vi "VL53L0X_PerformRefCalibration.vi"(11 "REV2mDistanceSensorDevRef":T1) -> (1 "PhaseCal":u8, 2 "VhvSettings":u8, 3 "REV2mDistanceSensorDevRef Out":T1)   [LabVIEW 2019, in "DistanceSensorDriver.lvlib"]
uses:
  DistanceSensorDriver.lvlib
  Typedef/REV2mDistanceSensorDevRef.ctl
  Typedef/Ports.ctl
panel:
  in  "PhaseCal":u8
  in  "VhvSettings":u8
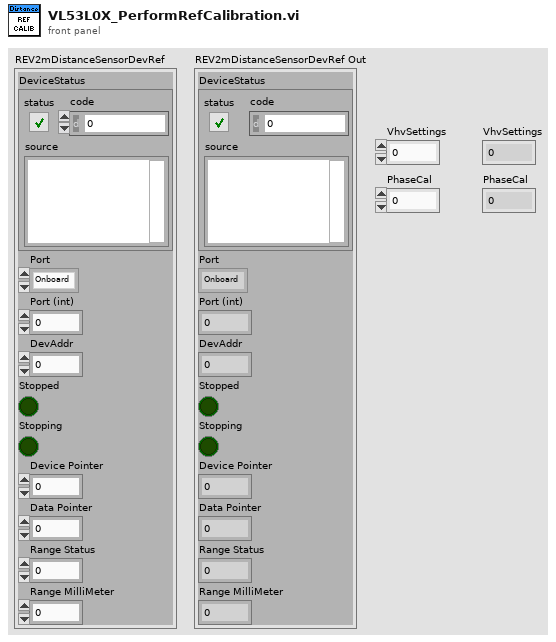
[diagram p1: front panel]
types:
  T1 = typedef "DistanceSensorDriver.lvlib/REV2mDistanceSensorDevRef.ctl" = cluster{"DeviceStatus":errorcluster, "Port":T2, "Port (int)":i32, "DevAddr":i32, "Stopped":bool, "Stopping":bool, "Device Pointer":u64, "Data Pointer":u64, "Range Status":u8, "Range MilliMeter":u16}
  T2 = typedef "DistanceSensorDriver.lvlib/Ports.ctl" = enum32{"Onboard", "MXP"}
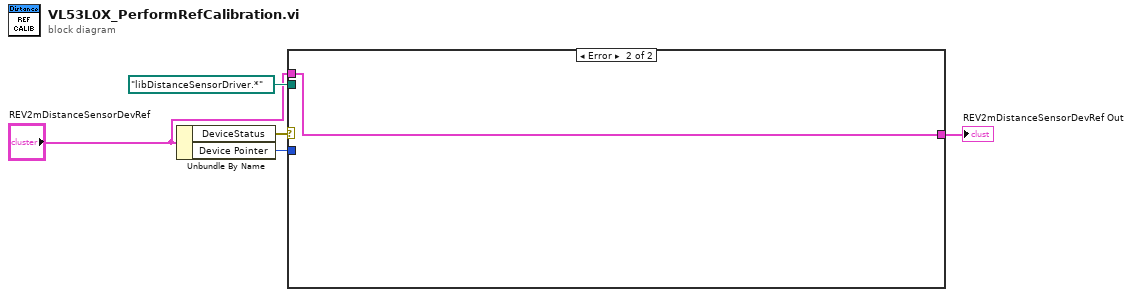
[diagram p0: block diagram]
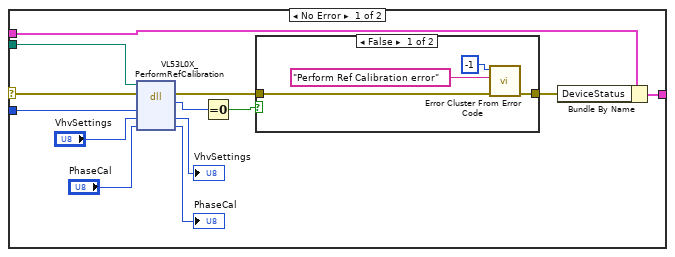
[diagram p2: hidden frame]
diagram:
  n1 = Unbundle By Name("REV2mDistanceSensorDevRef") -> ("DeviceStatus"=w1:errorcluster, "Device Pointer"=w4:u64)
  n2 = case shown="Error" w1 {
    selector: w1 -> [w6 _]
    tunnel: path "libDistanceSensorDriver.*" ("path in") -> [w16 _]
    tunnel: w4 -> [w13 _]
    tunnel: [w12 w24] -> w3
    tunnel: "REV2mDistanceSensorDevRef" -> [w11 w24]
    frame No Error {
      n3 = dll-call lib="?" fn="VL53L0X_PerformRefCalibration"(path in=w16, error in=w6, "Dev"=w13, "VhvSettings"="VhvSettings", "PhaseCal"="PhaseCal") -> (error out=w14:errorcluster, "Status"=w15:i32, "VhvSettings"=→"VhvSettings":u8, "PhaseCal"=→"PhaseCal":u8)  [unwired: 2 in, 1 out]
      n4 = Equal To 0?(x=w15) -> (x = 0?=w18:bool)
      n5 = case shown="False" w18 {
        tunnel: w14 -> [w19 w23]
        tunnel: [w22 w23] -> w17
        frame False {
          n6 = call <vilib>:"Error Cluster From Error Code.vi"("error in (no error)"=w19, "error message (\"\")"="Perform Ref Calibration error" ("error message (\"\")"), "error code (0)"=-1) -> ("error out"=w22:errorcluster)  [unwired: 6 in]
        }
        frame True {
        }
      }
      n7 = Bundle By Name(cluster=w11, "DeviceStatus"=w17) -> (w12:T1)
    }
    frame Error {
    }
  }
  "REV2mDistanceSensorDevRef Out" <- w3
